vi "Set Version.vi"(7 "Index":i32, 8 "error in":errorcluster, 10 "Build Version":T1, 11 "Builder in":refnum<class "Builder.lvclass">) -> (0 "error out":errorcluster, 3 "Builder out":refnum<class "Builder.lvclass">)   [LabVIEW 2021, in "App-Builder Library.lvlib" / "Builder.lvclass"]
uses:
  Builder.lvclass
  Builder.lvclass/Builder.ctl
  <vilib>/AppBuilder/AB_API_Simple/NI_App_Builder_API.lvlib
  <vilib>/AppBuilder/AB_API_Simple/Set Build Specification Version (path).vi
  <vilib>/AppBuilder/AB_API_Simple/Build Specification Version.ctl
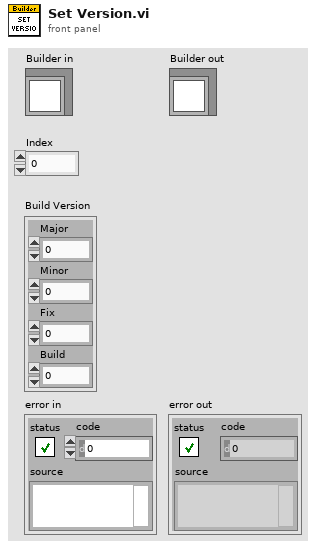
[diagram p1: front panel]
types:
  T1 = typedef "NI_App_Builder_API.lvlib/Build Specification Version.ctl" = cluster{"Major":u16, "Minor":u16, "Fix":u16, "Build":u16}
  T2 = typedef "App-Builder Library.lvlib/Builder.lvclass/Build specification.ctl" = cluster{"target name":string, "Build specification":string, "Project Path":path, "Build Object type":T3}
  T3 = typedef "App-Builder Library.lvlib/Builder.lvclass/Build object type.ctl" = enum16{"EXE", "RT EXE", "Deployable Packed"}
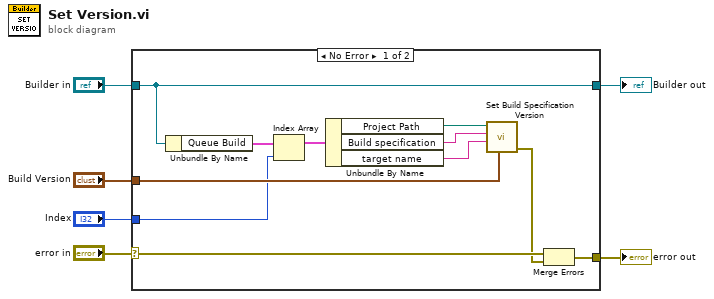
[diagram p0: block diagram]
diagram:
  n1 = case shown="No Error" "error in" {
    selector: "error in" -> [w17 w19]
    tunnel: [w14 w19] -> w5
    tunnel: [w15 w18] -> w3
    tunnel: "Builder in" -> [w15 w18]
    tunnel: "Build Version" -> [w16 _]
    tunnel: "Index" -> [w7 _]
    frame No Error {
      n2 = Unbundle By Name(w15) -> ("Queue Build"=w12:T2[])
      n3 = Index Array(array=w12, index=w7) -> (element=w8:T2)
      n4 = Unbundle By Name(w8) -> ("Project Path"=w11:path, "Build specification"=w9:string, "target name"=w10:string)
      n5 = call-poly <vilib>:"Set Build Specification Version.vi"("Build Specification Version"=w16, "Name of target (My Computer)"=w10, "Name of build specification"=w9, "Path to project"=w11) -> ("error out"=w13:errorcluster)  [unwired: 7 in]
      n6 = Merge Errors(w17, w13) -> (w14:errorcluster)
    }
    frame Error {
    }
  }
  "error out" <- w5
  "Builder out" <- w3
